vi "finishPrepareDoublePassPlay.vi"(8 "error in (no error)":errorcluster, 9 "OffensiveTeam in":refnum<class "Ally.lvclass">, 10 "Game":refnum<class "Game.lvclass">, 11 "PrepareDoublePassPlay in":refnum<class "PrepareDoublePassPlay.lvclass">) -> (0 "error out":errorcluster, 1 "OffensiveTeam out":refnum<class "Ally.lvclass">, 2 "FinishPrepareDoublePass?":bool, 3 "PrepareDoublePassPlay out":refnum<class "PrepareDoublePassPlay.lvclass">)   [LabVIEW 2023, in "PrepareDoublePassPlay.lvclass"]
uses:
  PrepareDoublePassPlay.lvclass
  Game_class/Game.lvclass
  Ally_class/Ally.lvclass
  C:/Users/ebert/Desktop/roboime/SSL_AI/Team_class/Team.lvclass
  Referee_class/command_interpreted.ctl
  Game_class/Game.lvclass/Game.ctl
  Team_class/Team.lvclass/Team.ctl
  Referee_class/Referee.lvclass/Referee.ctl
  Events_class/Events.lvclass/Events.ctl
  Ally_class/Ally.lvclass/Ally.ctl
  Ally_class/Read PreparePassPlaysEnum.vi
  Ally_class/Write PreparePassPlaysEnum.vi
  Game_class/Read EventsRef.vi
  Events_class/Read ball_out.vi
  Game_class/Read Referee.vi
  Referee_class/Read command_interpreted.vi
  Game_class/Read OffensiveTeam.vi
  Team_class/Read OffensivePlay Finished.vi
  Referee_class/Referee.lvclass
  Events_class/Events.lvclass
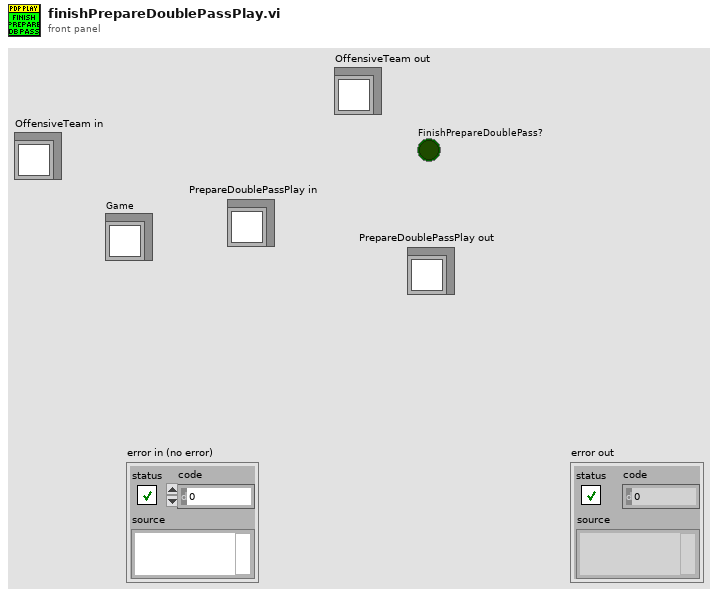
[diagram p1: front panel]
types:
  T1 = typedef "command_interpreted.ctl" = enum16{"Goal Ally", "Goal Enemy", "Ball Placement Enemy", "Ball Placement Ally", "Normal Half Time", "Extra Time  Break", "Extra Half Time", "None", "Post Game", "PKA Normal Start", "Prepare Kickoff Ally", "PKE Normal Start", "Prepare Kickoff Enemy", "Force Start", "Halt", "Timeout", "Prepare Penalty Ally", "Prepare Penalty Enemy", "PPA NormalStart", "PPE Normal Start", "Indirect Free Ally", "Direct Free Enemy", "Direct Free Ally", "Indirect Free Enemy", "Stop"}
  T2 = typedef "OffensivePlay.ctl" = enum16{"5RobotsPassGamePlay", "5PreparePassGame", "5RobotsKeeperGame", "KeeperPassToStriker", "5RobotsNormalGamePlay", "PrepareKeeperPass", "ACBPass", "ABCPass", "PrepareTriplePass", "TableWithStriker", "TableWith2ndStrikerPlay", "PrepareDoublePass", "PrepareRollToPass", "SimplePass", "PreparePass", "PassToStriker", "BallOutOfField", "PassTo2ndStriker", "StopOffensive", "Prepare Penalty Enemy", "EnemyPossessionAtEnemyField", "EnemyPossesionAtOurField", "TestPlay", "PreparePenaltyAlly", "KickPenaltyAlly", "PrepareKickoffAlly", "PrepareKickoffEnemy", "IndirectEnemy", "DirectEnemy", "PreparePassInGame1", "NormalGame", "DirectKick", "Pass", "Halt", "Timeout", "PassPlay", "PenaltyEnemy"}
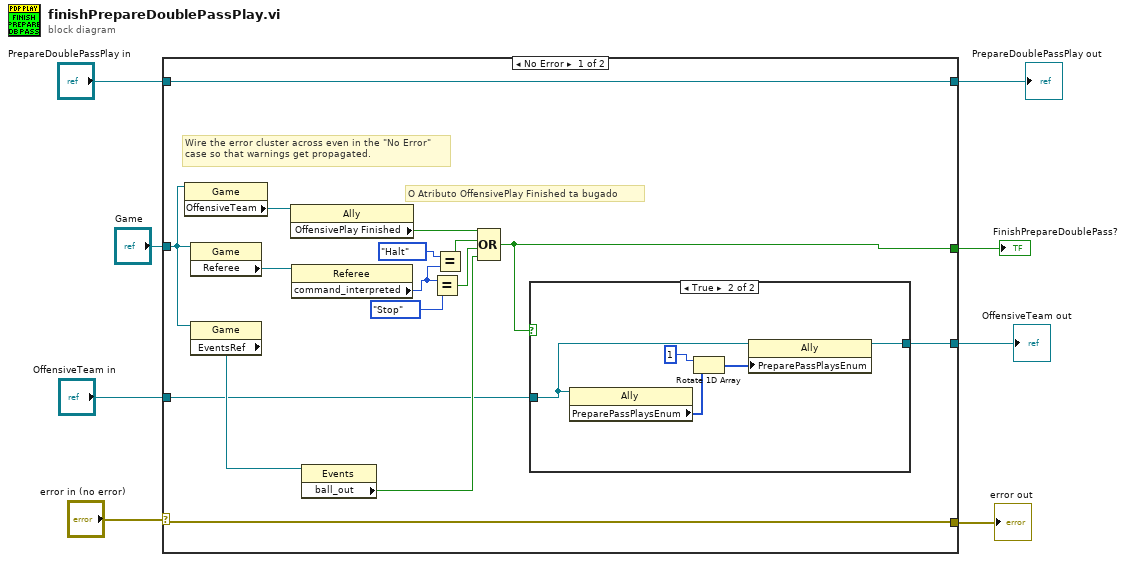
[diagram p0: block diagram]
diagram:
  n1 = case shown="No Error" "error in (no error)" {
    selector: "error in (no error)" -> [w23 w32]
    tunnel: [w23 w32] -> w7
    tunnel: [w24 w31] -> w4
    tunnel: "PrepareDoublePassPlay in" -> [w24 w31]
    tunnel: "Game" -> [w20 _]
    tunnel: [w11 _] -> w5
    tunnel: [w10 _] -> w2
    tunnel: "OffensiveTeam in" -> [w9 _]
    frame No Error {
      # "O Atributo OffensivePlay Finished ta bugado"
      # "Wire the error cluster across even in the \"No Error\"\ncase so that warnings get propagated."
      n2 = property class="Game"(reference=w20) -> ("OffensiveTeam"=w22:refnum<class "Ally.lvclass">)  [unwired: 1 in, 2 out]
      n3 = property class="Game"(reference=w20) -> ("Referee"=w21:refnum<class "Referee.lvclass">)  [unwired: 1 in, 2 out]
      n4 = property class="Game"(reference=w20) -> ("EventsRef"=w19:refnum<class "Events.lvclass">)  [unwired: 1 in, 2 out]
      n5 = property class="Ally"(reference=w22) -> ("OffensivePlay Finished"=w12:bool)  [unwired: 1 in, 2 out]
      n6 = property class="Referee"(reference=w21) -> ("command_interpreted"=w16:T1)  [unwired: 1 in, 2 out]
      n7 = property class="Events"(reference=w19) -> ("ball_out"=w13:bool)  [unwired: 1 in, 2 out]
      n8 = Equal?(x=w16, y=command_interpreted."Stop") -> (x = y?=w18:bool)
      n9 = Equal?(x=command_interpreted."Halt" ("y"), y=w16) -> (x = y?=w14:bool)
      n10 = Compound Arithmetic op=OR(w12, w14, w18, w13) -> (w11:bool)
      n11 = case shown="True" w11 {
        tunnel: [w25 w28] -> w10
        tunnel: w9 -> [w25 w27]
        frame False {
        }
        frame True {
          n12 = property class="Ally"(reference=w27) -> ("PreparePassPlaysEnum"=w26:T2[])  [unwired: 1 in, 2 out]
          n13 = Rotate 1D Array(1:w26, 2:1 ("n")) -> (0:w29:T2[])
          n14 = property class="Ally"(reference=w27, "PreparePassPlaysEnum"=w29) -> (reference out=w28:refnum<class "Ally.lvclass">)  [unwired: 1 in, 1 out]
        }
      }
    }
    frame Error {
    }
  }
  "error out" <- w7
  "FinishPrepareDoublePass?" <- w5
  "PrepareDoublePassPlay out" <- w4
  "OffensiveTeam out" <- w2
